vi "Check String Type.vi"(8 "error in (no error)":errorcluster, 10 "String":string, 11 "Value Type in":refnum<class "Value Type.lvclass">) -> (0 "error out":errorcluster, 3 "Value Type out":refnum<class "Value Type.lvclass">)   [LabVIEW 2020, in "Composed Columns.lvlib" / "Value Type.lvclass"]
uses:
  Value Type.lvclass
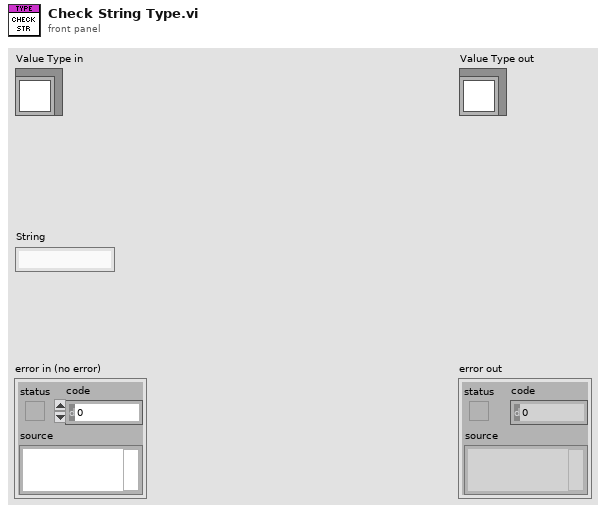
[diagram p1: front panel]
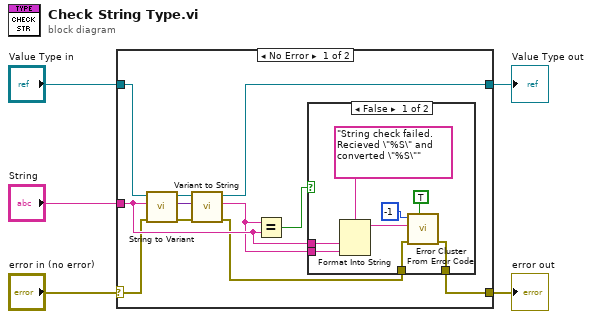
[diagram p0: block diagram]
diagram:
  n1 = case shown="No Error" "error in (no error)" {
    selector: "error in (no error)" -> [w8 w27]
    tunnel: [w9 w27] -> w4
    tunnel: [w14 w26] -> w2
    tunnel: "Value Type in" -> [w16 w26]
    tunnel: "String" -> [w11 _]
    frame No Error {
      n2 = call-dynamic "String to Variant.vi"("error in (no error)"=w8, "String"=w11, "Value Type in"=w16) -> ("error out"=w7:errorcluster, "Variant"=w13:variant, "Value Type out"=w15:refnum<class "Value Type.lvclass">)  [unwired: 6 in]
      n3 = call-dynamic "Variant to String.vi"("error in (no error)"=w7, "Variant"=w13, "Value Type in"=w15) -> ("error out"=w6:errorcluster, "String"=w10:string, "Value Type out"=w14:refnum<class "Value Type.lvclass">)  [unwired: 6 in]
      n4 = Equal?(x=w10, y=w11) -> (x = y?=w12:bool)
      n5 = case shown="False" w12 {
        tunnel: w11 -> [w23 _]
        tunnel: w10 -> [w22 _]
        tunnel: [w19 w25] -> w9
        tunnel: w6 -> [w18 w25]
        frame False {
          n6 = Format Into String(format string="String check failed. Recieved \"%S\" and converted \"%S\"", w23, w22) -> (resulting string=w20:string)  [unwired: 2 in, 1 out]
          n7 = call <vilib>:"Error Cluster From Error Code.vi"("show call chain? (False)"=TRUE, "error in (no error)"=w18, "error message (\"\")"=w20, "error code (0)"=-1) -> ("error out"=w19:errorcluster)  [unwired: 5 in]
        }
        frame True {
        }
      }
    }
    frame Error {
    }
  }
  "error out" <- w4
  "Value Type out" <- w2
